vi "WebStartup.vi"(6 "LabVIEW Web Service":refnum<class "Web Service.lvclass">) -> ()   [LabVIEW 2015]
uses:
  <vilib>/wsapi/Web Service.lvclass
  TypeDef/RoomsActionEnum.ctl
  TypeDef/PersonnelActions.ctl
panel:
  out "Data Out":string
  out "error out":errorcluster
  # "Use the web service input terminal to call the VIs on the Service subpalette of the Web Services palette. Do not remove it from the connector pane unless you don't need access to the palette."
  # "Any additional terminals added to the connector pane of a startup VI will be ignored."
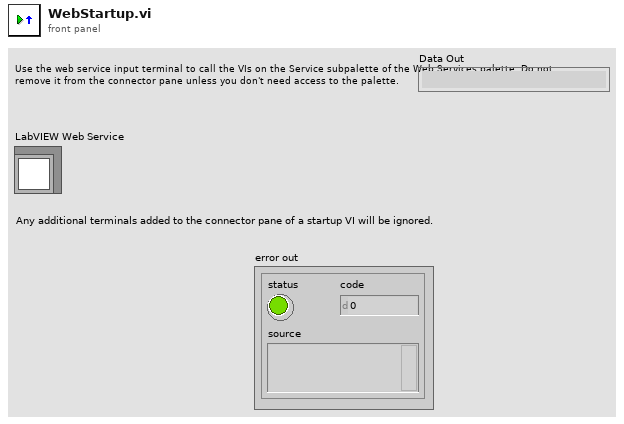
[diagram p1: front panel]
types:
  T1 = typedef "PersonnelActions.ctl" = enum16{"Init", "Read Personnel", "Add Personnel", "Remove Personnel", "Read Name", "Write Name", "Read Role", "Write Role", "Read Requests", "Add Requests", "Remove Requests", "Read PUIDs"}
  T2 = typedef "RoomsActionEnum.ctl" = enum16{"Init", "Add Room", "Remove Room", "Read Room", "Read Flag", "Read Flag State", "Write Flag State", "Read Flag Color", "Write Flag Color", "Read Bed Vacant", "Write Bed Vacant", "Read Personnel", "Add Personnel", "Remove Personnel", "Read Requests", "Add Request", "Remove Request", "Read Beacon ID", "Write Beacon ID", "Write Bed URL", "Read Bed URL", "Read Rooms Numbers", "Write Flag"}
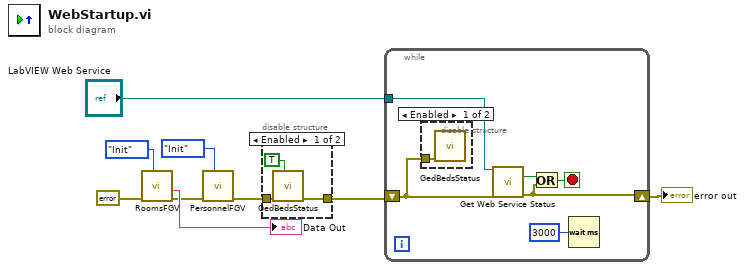
[diagram p0: block diagram]
diagram:
  n1 = call "RoomsFGV.vi"("Actions"=RoomsActionEnum."Init", "error in (no error)"=errorcluster {"status"=FALSE, "code"=0, "source"=""} ("error constant")) -> ("error out"=w3:errorcluster, "Data Out"=→"Data Out":string)  [unwired: 8 in]
  n2 = call "PersonnelFGV.vi"("Actions"=PersonnelActions."Init", "error in (no error)"=w3) -> ("error out"=w2:errorcluster)  [unwired: 8 in, 1 out]
  n3 = disable-structure shown="Enabled" {
    disable-tunnel: w2 -> [w11 _]
    disable-tunnel: [w10 _] -> w6
    frame Enabled {
      n4 = call "GedBedsStatus.vi"("Initialize"=TRUE, "error in (no error)"=w11) -> ("error out"=w10:errorcluster)  [unwired: 9 in]
    }
    frame Disabled {
    }
  }
  n5 = while {
    tunnel: "LabVIEW Web Service" -> [w17]
    shift-right: [w15] -> w8
    shift-left: w6 -> [w13]
    stop <- w16 stop-if-true
    n6 = disable-structure shown="Enabled" {
      disable-tunnel: w13 -> [w19 _]
      frame Enabled {
        n7 = call "GedBedsStatus.vi"("error in (no error)"=w19) -> ()  [unwired: 10 in, 1 out]
      }
      frame Disabled {
      }
    }
    n8 = call <vilib>:"Get Web Service Status.vi"("LabVIEW Web Service"=w17, "error in (no error)"=w13) -> ("service stopping?"=w18:bool, "error out"=w15:errorcluster)  [unwired: 11 in, 1 out]
    n9 = Or(x=w18, y=w15) -> (x .or. y?=w16:bool)
    n10 = Wait (ms)(milliseconds to wait=u32 3000) -> ()  [unwired: 1 out]
  }
  "error out" <- w8
